vi "IBM4_Read(I1).vi"(8 "error in":errorcluster, 10 "Channel":i32, 11 "COM resource in":refnum<visa-resource-name>="COM9") -> (0 "error out":errorcluster, 2 "output":i32, 3 "COM resource out":refnum<visa-resource-name>)   [LabVIEW 2021, in "IBM4.lvlib"]
doc: "This VI interfaces with the IBM4 to perform a read operation.\n\nThe input channel must be between 0 and 3, while the output will in binary format (thus, integer).\nOnly a single read operation is made with this VI. \n\nAlternate read operations exist covering binary or floating point, single reading, multiple readings, and an average of multiple readings (floating point only)."
uses:
  <instrlib>/IBM4/IBM4.lvlib
panel:
  out "read buffer":string
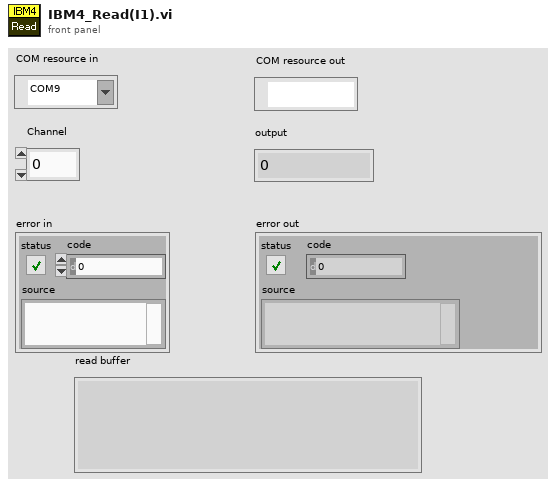
[diagram p1: front panel]
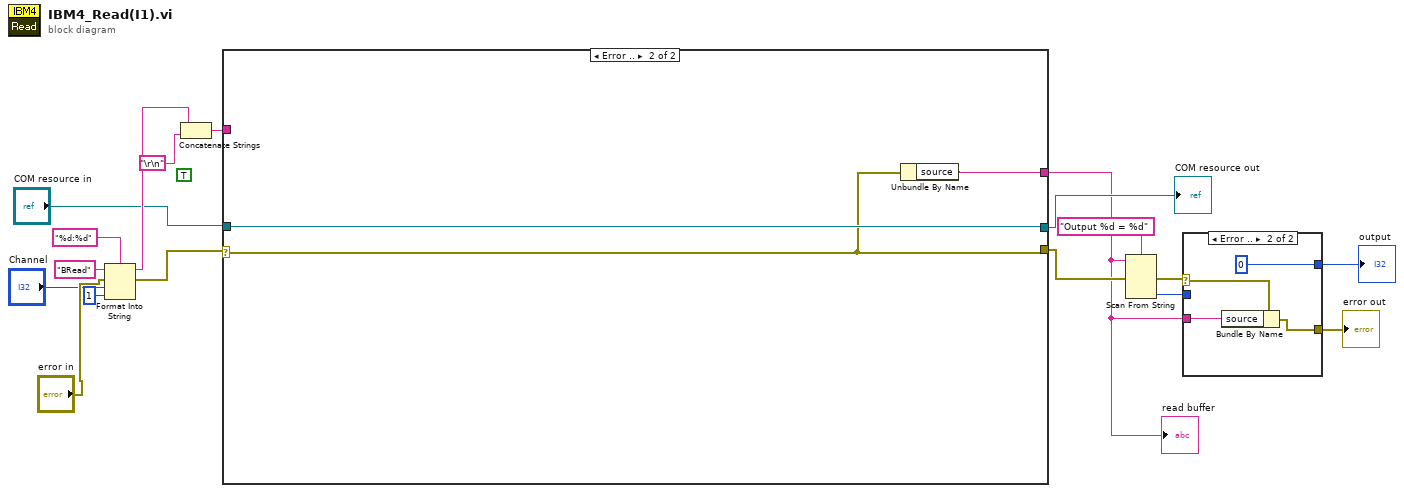
[diagram p0: block diagram]
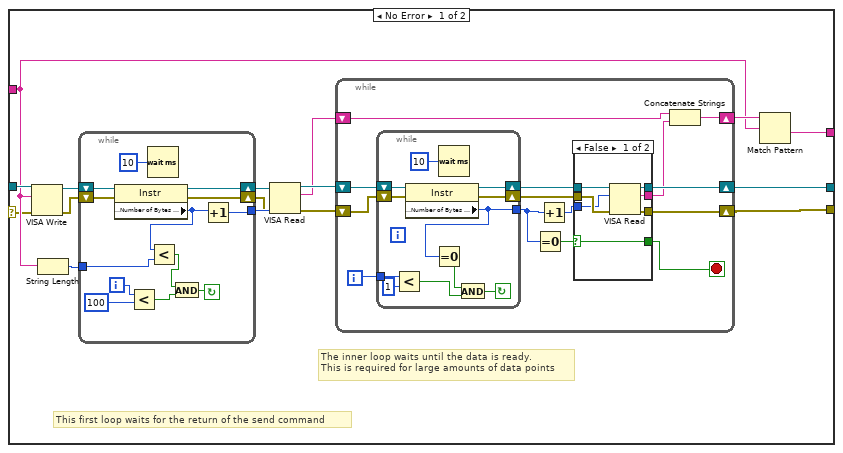
[diagram p3: hidden frame]
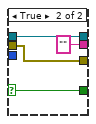
[diagram p4: hidden frame]
diagram:
  (unwired) TRUE ("Enable Termination\nChar (T)")
  n1 = Format Into String(format string="%d:%d", initial string="BRead", error in="error in", "Channel", 1 ("input 2")) -> (resulting string=w9:string, error out=w1:errorcluster)
  n2 = Concatenate Strings(w9, "\r\n") -> (w8:string)
  n3 = case shown="Error .." w1 {
    selector: w1 -> [w21 w84]
    tunnel: "COM resource in" -> [w34 w86]
    tunnel: [w20 w84] -> w12
    tunnel: [w32 w85] -> w3
    tunnel: w8 -> [w31 _]
    tunnel: [w19 w86] -> w13
    frame No Error {
      # "The inner loop waits until the data is ready.\nThis is required for large amounts of data points"
      # "This first loop waits for the return of the send command"
      n4 = VISA Write(VISA resource name=w34, write buffer=w31, error in (no error)=w21) -> (VISA resource name out=w30:refnum<visa-resource-name>, error out=w29:errorcluster)  [unwired: 1 out]
      n5 = String Length(string=w31) -> (length=w22:i32)
      n6 = while {
        tunnel: [w36] -> w27
        shift-right: [w46] -> w28
        shift-left: w30 -> [w47]
        shift-right: [w44] -> w26
        shift-left: w29 -> [w45]
        tunnel: w22 -> [w42]
        i -> [w37]
        stop <- w40 continue-if-true
        n7 = property class="Instr"(reference=w47, error in=w45) -> (reference out=w46:refnum<visa-resource-name>, error out=w44:errorcluster, "Serial Settings:Number of Bytes at Serial Port"=w35:u32)
        n8 = Less?(x=w37, y=100) -> (x < y?=w39:bool)
        n9 = Wait (ms)(milliseconds to wait=u32 10) -> ()  [unwired: 1 out]
        n10 = Less?(x=w35, y=w42) -> (x < y?=w38:bool)
        n11 = And(x=w38, y=w39) -> (x .and. y?=w40:bool)
        n12 = Increment(x=w35) -> (x+1=w36:u32)
      }
      n13 = VISA Read(VISA resource name=w28, byte count=w27, error in (no error)=w26) -> (VISA resource name out=w25:refnum<visa-resource-name>, read buffer=w23:string, error out=w24:errorcluster)  [unwired: 1 out]
      n14 = while {
        shift-right: [w61] -> w19
        shift-left: w25 -> [w59]
        shift-right: [w60] -> w20
        shift-left: w24 -> [w57]
        shift-right: [w55] -> w33
        shift-left: w23 -> [w53]
        i -> [w52]
        stop <- w48 stop-if-true
        n15 = while {
          tunnel: [w78] -> w51
          shift-right: [w82] -> w58
          shift-left: w59 -> [w83]
          shift-right: [w80] -> w56
          shift-left: w57 -> [w81]
          tunnel: w52 -> [w77]
          stop <- w75 continue-if-true
          n16 = Less?(x=w77, y=1) -> (x < y?=w74:bool)
          n17 = property class="Instr"(reference=w83, error in=w81) -> (reference out=w82:refnum<visa-resource-name>, error out=w80:errorcluster, "Serial Settings:Number of Bytes at Serial Port"=w78:u32)
          n18 = Equal To 0?(x=w78) -> (x = 0?=w73:bool)
          n19 = Wait (ms)(milliseconds to wait=u32 10) -> ()  [unwired: 1 out]
          n20 = And(x=w73, y=w74) -> (x .and. y?=w75:bool)
        }
        n21 = Equal To 0?(x=w51) -> (x = 0?=w49:bool)
        n22 = Increment(x=w51) -> (x+1=w50:u32)
        n23 = case shown="False" w49 {
          selector: w49 -> [w62 w71]
          tunnel: [w68 w72] -> w61
          tunnel: [w67 w70] -> w60
          tunnel: w58 -> [w66 w72]
          tunnel: w56 -> [w65 w70]
          tunnel: [w64 "" ("read buffer")] -> w54
          tunnel: w50 -> [w63 _]
          tunnel: [w62 w71] -> w48
          frame False {
            n24 = VISA Read(VISA resource name=w66, byte count=w63, error in (no error)=w65) -> (VISA resource name out=w68:refnum<visa-resource-name>, read buffer=w64:string, error out=w67:errorcluster)  [unwired: 1 out]
          }
          frame True {
          }
        }
        n25 = Concatenate Strings(w53, w54) -> (w55:string)
      }
      n26 = Match Pattern(string=w33, regular expression=w31) -> (after substring=w32:string)  [unwired: 1 in, 3 out]
    }
    frame Error {
      n27 = Unbundle By Name(w84) -> ("source"=w85:string)
    }
  }
  "COM resource out" <- w13
  "read buffer" <- w3
  n28 = Scan From String(format string="Output %d = %d", input string=w3, error in=w12) -> (error out=w7:errorcluster, output 2=w6:i32)  [unwired: 4 in, 2 out]
  n29 = case shown="Error .." w7 {
    selector: w7 -> [w87 w91]
    tunnel: w6 -> [w88 _]
    tunnel: [w88 0] -> w5
    tunnel: [w87 w89] -> w4
    tunnel: w3 -> [_ w90]
    frame No Error {
    }
    frame Error {
      n30 = Bundle By Name(cluster=w91, "source"=w90) -> (w89:errorcluster)
    }
  }
  "error out" <- w4
  "output" <- w5
